vi "Default Settings.vi"(4 "Font ComboBox":refnum<vi>, 6 "VI":refnum<vi>, 8 "error in":errorcluster, 11 "INI Settings in":refnum<class "INI Settings.lvclass">) -> (0 "error out":errorcluster, 3 "INI Settings out":refnum<class "INI Settings.lvclass">)   [LabVIEW 2020, in "INI Settings.lvclass"]
doc: "Tests the default settings by first removing the keys from the LabVIEW.ini file and then reading the settings."
uses:
  INI Settings.lvclass
  INI Settings.lvclass/INI Settings.ctl
  a9744b65-5dfe-4034-b049-38d610e378a7.vi
  vi.lib/LabVIEW Icon API/lv_icon/lv_icon.lvlib
  resource/plugins/NIIconEditor/Controls/Tools.ctl
  vi.lib/LabVIEW Icon API/lv_icon/Controls/IEColor.ctl
  vi.lib/LabVIEW Icon API/lv_icon/Controls/Alignment.ctl
  vi.lib/LabVIEW Icon API/lv_icon/Controls/Font.ctl
  vi.lib/LabVIEW Icon API/lv_icon/Controls/BodyText.ctl
  resource/plugins/NIIconEditor/Controls/Font Size.ctl
  resource/plugins/NIIconEditor/INI/INI Data.ctl
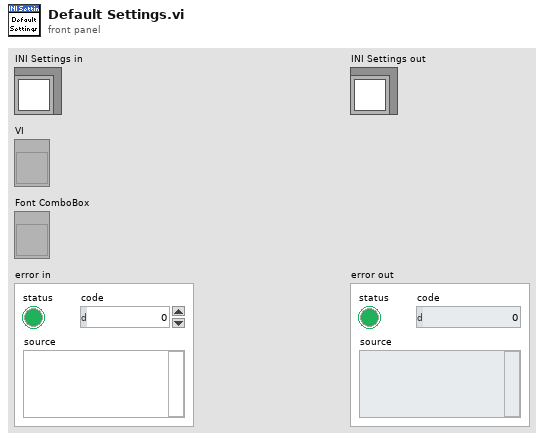
[diagram p1: front panel]
types:
  T1 = typedef "lv_icon.lvlib/INI Data.ctl" = cluster{"Show Terminals?":bool, "Text":cluster{"Font":T2, "Alignment":T3, "Size":T4}, "3rd party Templates":cluster{"Store 3rd party Templates?":bool, "Folder Name":string}, "Merge user layers on commit":bool, "Body Text":T5, "Fill Color":T6, "Edge Color":T6, "Tab":u16, "Tool":T7, "Disable Layers?":bool}
  T2 = typedef "Font.ctl" = string
  T3 = typedef "Alignment.ctl" = u16
  T4 = typedef "Font Size.ctl" = u8
  T5 = typedef "BodyText.ctl" = cluster{"Line 1 text":string, "Line 2 text":string, "Line 3 text":string, "Line 4 text":string, "Line 1 color":u32, "Line 2 color":u32, "Line 3 color":u32, "Line 4 color":u32, "Body Text Spec":cluster{"Font":T2, "Alignment":T3, "Size":u8}, "Center text vertically":bool, "Capitalize Text":bool}
  T6 = typedef "IEColor.ctl" = u32
  T7 = typedef "Tools.ctl" = enum32{"Pencil", "Line", "Dropper", "Fill", "Rectangle", "Filled Rectangle", "Ellipse", "Filled Ellipse", "Eraser", "Text", "Select", "Move"}
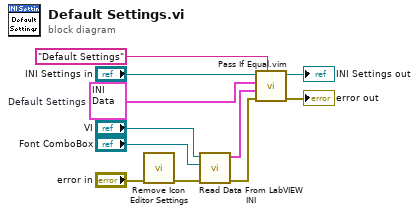
[diagram p0: block diagram]
diagram:
  w1 = T1 {"Show Terminals?"=FALSE, "Text"={"Font"="Small Fonts", "Alignment"=1, "Size"=9}, "3rd party Templates"={"Store 3rd party Templates?"=TRUE, "Folder Name"="3rd party"}, "Merge user layers on commit"=FALSE, "Body Text"={"Line 1 text"="", "Line 2 text"="", "Line 3 text"="", "Line 4 text"="", "Line 1 color"=0, "Line 2 color"=0, "Line 3 color"=0, "Line 4 color"=0, "Body Text Spec"={"Font"="Small Fonts", "Alignment"=1, "Size"=9}, "Center text vertically"=TRUE, "Capitalize Text"=TRUE}, "Fill Color"=16711680, "Edge Color"=0, "Tab"=0, "Tool"=enum."Pencil", "Disable Layers?"=FALSE}  # Default Settings
  n1 = call "Remove Icon Editor Settings.vi"("error in"="error in") -> ("error out"=w10:errorcluster)  [unwired: 10 in]
  n2 = call "Read Data From LabVIEW INI.vi"("error in"=w10, "DNL_Font"="Font ComboBox", "IE VI Ref"="VI") -> ("error out"=w11:errorcluster, "INI Data"=w5:T1)  [unwired: 7 in]
  n3 = call "Pass If Equal.vim"("Description"="Default Settings", "error in (no error)"=w11, "Actual"=w5, "Expected"=w1, "LUnit Test Case In"="INI Settings in") -> ("error out"=→"error out":errorcluster, "LUnit Test Case Out"=→"INI Settings out":refnum<class "INI Settings.lvclass">)  [unwired: 5 in]
